vi "GPIB Set Timeout.vi"(4 "Error In":errorcluster, 6 "Timeout":u32, 7 "VISA resource name":refnum<visa-resource-name>) -> (0 "Error Out":errorcluster, 2 "Old Timeout":u32, 3 "dup VISA resource name":refnum<visa-resource-name>)   [LabVIEW 2024]
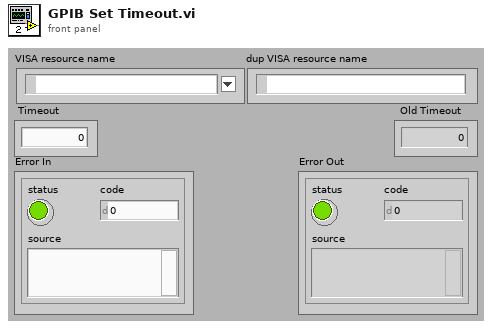
[diagram p1: front panel]
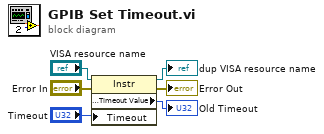
[diagram p0: block diagram]
diagram:
  n1 = property class="Instr"(reference="VISA resource name", error in="Error In", "Timeout"="Timeout") -> (reference out=→"dup VISA resource name":refnum<visa-resource-name>, error out=→"Error Out":errorcluster, "General Settings:Timeout Value"=→"Old Timeout":u32)
